vi "Init.vi"(11 "error in (no error)":errorcluster) -> (4 "FPGA API out":refnum<class "FPGA API Mock.lvclass">, 15 "error out":errorcluster)   [LabVIEW 2019, in "FPGA API Mock.lvclass"]
uses:
  FPGA API Mock.lvclass
  FPGA/TypeDef/DO index.ctl
  Data.ctl
  FPGA API Mock.lvclass/FPGA API Mock.ctl
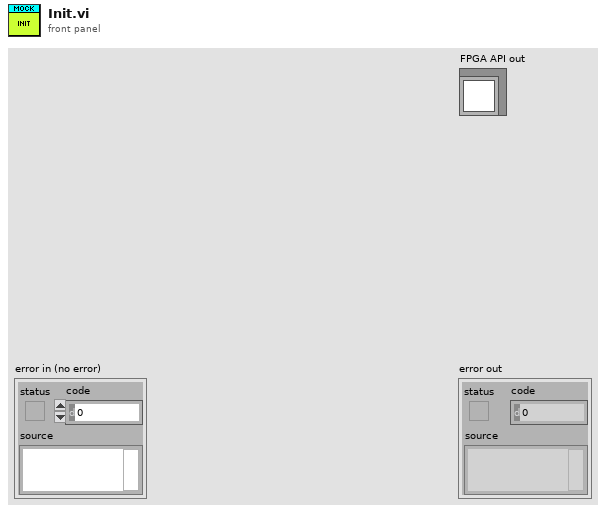
[diagram p1: front panel]
types:
  T1 = typedef "FPGA API Mock.lvclass/Data.ctl" = cluster{"DO":bool[], "DI":bool[], "AI":dbl[], "AO":dbl[]}
  T2 = typedef "DO index.ctl" = u8
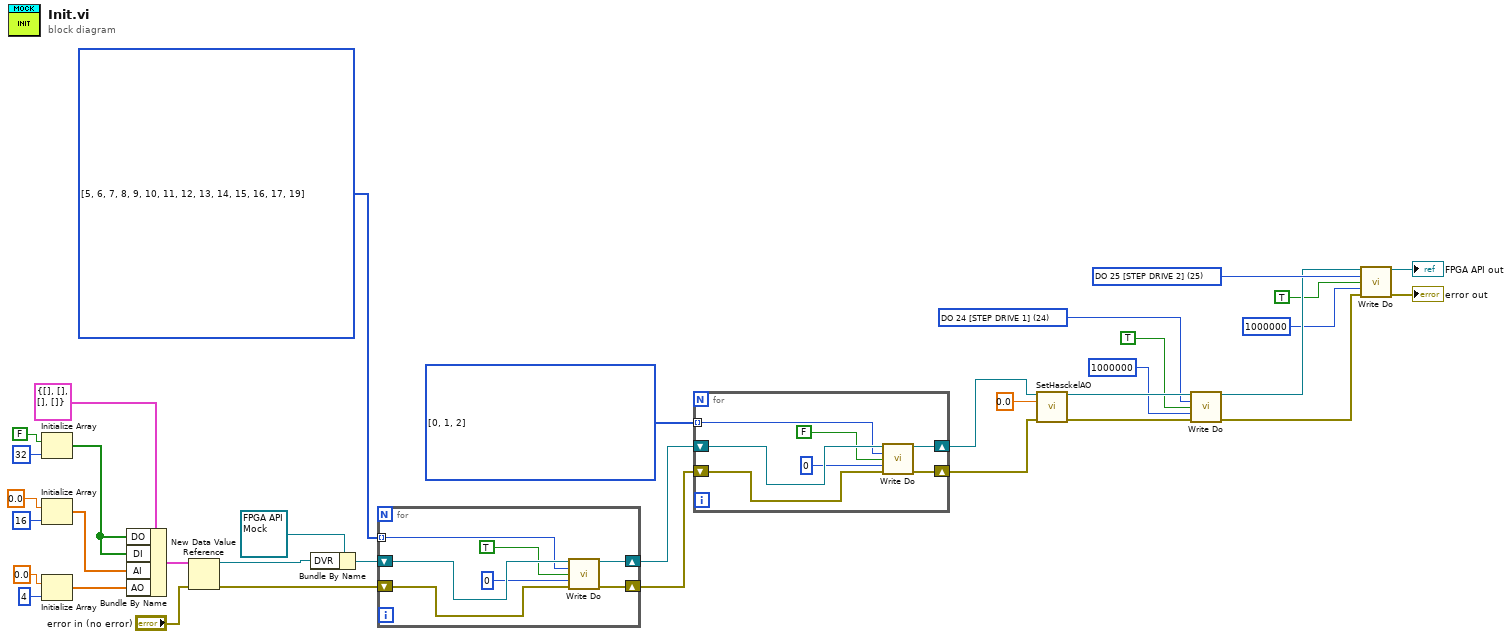
[diagram p0: block diagram]
diagram:
  w21 = T2[] [0, 1, 2] items=["DO 0 [KP1] [M12]", "DO 1 [ON KP2] [M21]", "DO 2 [ON KP3] [M24]", "DO 3 [WATER Y18.1 [DO3]]", "DO 4 [WATER Y18.2 [DO4]]", "DO 5 [KP6 Y29.1 33.7]", "DO 6 [KP7 Y29.2 33.8]", "DO 7 [KP8 Y29.3 33.9]", "DO 8 [KP9 Y29.4  33.12]", "DO 9 [KP10 Y29.5 33.1]", "DO 10 [KP11 Y29.6 33.2]", "DO 11 [KP12 Y29.7  33.13]", "DO 12 [KP13 Y29.8  33.11]", "DO 13 [KP14 Y29.9 33.10]", "DO 14 [KP15 Y29.10  33.6]", "DO 15 [KP16 Y29.11  33.5]", "DO 16 [KP17 Y29.12  33.4]", "DO 17 [KP18 Y29.13 33.3]", "DO 18 [AIR KP19]", "DO 19 [STEP DRIVE EN KP20]", "DO 20 [KP21 Y44.1 OPEN]", "DO 21 [ KP22 Y44.1 CLOSE]", "DO 22 [ KP23 Y44.2 OPEN]", "DO 23", "DO 24 [STEP DRIVE 1]", "DO 25 [STEP DRIVE 2]"] ("#DO")
  w29 = T2 25 items=["DO 0 [KP1 [DO 0]]", "DO 1 [ON KP2 [DO 1]]", "DO 2 [ON KP3 [DO 2]]", "DO 3 [WATER Y18.1 [DO3]]", "DO 4 [WATER Y18.2 [DO4]]", "DO 5 [KP6 Y29.1 33.7]", "DO 6 [KP7 Y29.2 33.8]", "DO 7 [KP8 Y29.3 33.9]", "DO 8 [KP9 Y29.4  33.12]", "DO 9 [KP10 Y29.5 33.1]", "DO 10 [KP11 Y29.6 33.2]", "DO 11 [KP12 Y29.7  33.13]", "DO 12 [KP13 Y29.8  33.11]", "DO 13 [KP14 Y29.9 33.10]", "DO 14 [KP15 Y29.10  33.6]", "DO 15 [KP16 Y29.11  33.5]", "DO 16 [KP17 Y29.12  33.4]", "DO 17 [KP18 Y29.13 33.3]", "DO 18 [AIR KP19]", "DO 19 [STEP DRIVE EN KP20]", "DO 20 [KP21 Y44.1 OPEN]", "DO 21 [ KP22 Y44.1 CLOSE]", "DO 22 [ KP23 Y44.2 OPEN]", "DO 23", "DO 24 [STEP DRIVE 1]", "DO 25 [STEP DRIVE 2]"] ("#DO")
  w32 = T2 24 items=["DO 0 [KP1 [DO 0]]", "DO 1 [ON KP2 [DO 1]]", "DO 2 [ON KP3 [DO 2]]", "DO 3 [WATER Y18.1 [DO3]]", "DO 4 [WATER Y18.2 [DO4]]", "DO 5 [KP6 Y29.1 33.7]", "DO 6 [KP7 Y29.2 33.8]", "DO 7 [KP8 Y29.3 33.9]", "DO 8 [KP9 Y29.4  33.12]", "DO 9 [KP10 Y29.5 33.1]", "DO 10 [KP11 Y29.6 33.2]", "DO 11 [KP12 Y29.7  33.13]", "DO 12 [KP13 Y29.8  33.11]", "DO 13 [KP14 Y29.9 33.10]", "DO 14 [KP15 Y29.10  33.6]", "DO 15 [KP16 Y29.11  33.5]", "DO 16 [KP17 Y29.12  33.4]", "DO 17 [KP18 Y29.13 33.3]", "DO 18 [AIR KP19]", "DO 19 [STEP DRIVE EN KP20]", "DO 20 [KP21 Y44.1 OPEN]", "DO 21 [ KP22 Y44.1 CLOSE]", "DO 22 [ KP23 Y44.2 OPEN]", "DO 23", "DO 24 [STEP DRIVE 1]", "DO 25 [STEP DRIVE 2]"] ("#DO")
  w35 = T2[] [5, 6, 7, 8, 9, 10, 11, 12, 13, 14, 15, 16, 17, 19] items=["DO 0 [KP1 [DO 0]]", "DO 1 [ON KP2 [DO 1]]", "DO 2 [ON KP3 [DO 2]]", "DO 3 [WATER Y18.1 [DO3]]", "DO 4 [WATER Y18.2 [DO4]]", "DO 5 [KP6 Y29.1 33.7]", "DO 6 [KP7 Y29.2 33.8]", "DO 7 [KP8 Y29.3 33.9]", "DO 8 [KP9 Y29.4  33.12]", "DO 9 [KP10 Y29.5 33.1]", "DO 10 [KP11 Y29.6 33.2]", "DO 11 [KP12 Y29.7  33.13]", "DO 12 [KP13 Y29.8  33.11]", "DO 13 [KP14 Y29.9 33.10]", "DO 14 [KP15 Y29.10  33.6]", "DO 15 [KP16 Y29.11  33.5]", "DO 16 [KP17 Y29.12  33.4]", "DO 17 [KP18 Y29.13 33.3]", "DO 18 [AIR KP19]", "DO 19 [STEP DRIVE EN KP20]", "DO 20 [KP21 Y44.1 OPEN]", "DO 21 [ KP22 Y44.1 CLOSE]", "DO 22 [ KP23 Y44.2 OPEN]", "DO 23", "DO 24 [STEP DRIVE 1]", "DO 25 [STEP DRIVE 2]"] ("#DO")
  n1 = Initialize Array(FALSE ("value"), 32 ("dimension size")) -> (w8:bool[])
  n2 = Initialize Array(0.0 ("element"), 16 ("dimension size")) -> (w14:dbl[])
  n3 = Initialize Array(0.0 ("element"), 4 ("dimension size")) -> (w11:dbl[])
  n4 = Bundle By Name(cluster=T1 {"DO"=[], "DI"=[], "AI"=[], "AO"=[]} ("Data"), "DO"=w8, "DI"=w8, "AI"=w14, "AO"=w11) -> (w6:T1)
  n5 = New Data Value Reference(data value=w6, error in="error in (no error)") -> (data value reference=w4:refnum<data-value>, error out=w2:errorcluster)
  n6 = Bundle By Name(cluster=refnum<class "FPGA API Mock.lvclass"> refnum ("FPGA API in"), "DVR"=w4) -> (w1:refnum<class "FPGA API Mock.lvclass">)
  n7 = for {
    tunnel: w35 -> [w38] mode=indexing
    shift-right: [w41] -> w20
    shift-left: w1 -> [w42]
    shift-right: [w40] -> w18
    shift-left: w2 -> [w39]
    n8 = call-dynamic "Write Do.vi"("FPGA API in"=w42, "#DO"=w38, "value"=TRUE, "Time uSec"=u32 0, "error in (no error)"=w39) -> ("FPGA API out"=w41:refnum<class "FPGA API Mock.lvclass">, "error out"=w40:errorcluster)  [unwired: 9 in]
  }
  n9 = for {
    tunnel: w21 -> [w45] mode=indexing
    shift-right: [w48] -> w19
    shift-left: w20 -> [w49]
    shift-right: [w47] -> w17
    shift-left: w18 -> [w46]
    n10 = call-dynamic "Write Do.vi"("FPGA API in"=w49, "#DO"=w45, "value"=FALSE, "Time uSec"=u32 0, "error in (no error)"=w46) -> ("FPGA API out"=w48:refnum<class "FPGA API Mock.lvclass">, "error out"=w47:errorcluster)  [unwired: 9 in]
  }
  n11 = call-dynamic "SetHasckelAO.vi"("FPGA API in"=w19, "Haskel in"=0.0, "error in (no error)"=w17) -> ("FPGA API out"=w33:refnum<class "FPGA API Mock.lvclass">, "error out"=w25:errorcluster)  [unwired: 11 in]
  n12 = call-dynamic "Write Do.vi"("FPGA API in"=w33, "#DO"=w32, "value"=TRUE, "Time uSec"=u32 1000000, "error in (no error)"=w25) -> ("FPGA API out"=w28:refnum<class "FPGA API Mock.lvclass">, "error out"=w24:errorcluster)  [unwired: 9 in]
  n13 = call-dynamic "Write Do.vi"("FPGA API in"=w28, "#DO"=w29, "value"=TRUE, "Time uSec"=u32 1000000, "error in (no error)"=w24) -> ("FPGA API out"=→"FPGA API out":refnum<class "FPGA API Mock.lvclass">, "error out"=→"error out":errorcluster)  [unwired: 9 in]
